vi "Recloser2.vi"() -> ()   [LabVIEW 2016]
uses:
  <vilib>/Utility/error.llb/DialogType.ctl
  <vilib>/Analysis/3filter.llb/Filter Passband Type.ctl
  <vilib>/FPGAPlugInAG/cRIO-9039 (Sync)/niLvFpga_Open_cRIO-9039 (Sync).vi
  <vilib>/rvi/interface/common/dynamic/niFpgaDynamicAddResources.vi
  <vilib>/addons/Electrical Power/Basic/Measurement/RMS (N Channels).vi
  <vilib>/measure/matone.llb/Extract Single Tone Information N Chan.vi
  <vilib>/Analysis/3filter.llb/Butterworth Filter (DBL).vi
  <vilib>/Utility/error.llb/Error Cluster From Error Code.vi
  <vilib>/rvi/errors/niLvFpgaAdjustHostInterfaceError.vi
  <vilib>/FPGAPlugInAG/Dynamic/niLvFpga_Abort_Dynamic.vi
  <vilib>/FPGAPlugInAG/Dynamic/niLvFpga_Close_Dynamic.vi
  <vilib>/rvi/interface/nirviOpenFPGA/nirviOpenFPGA.xnode
  FPGA Bitfiles/IntelliRupter2_FPGATarget.lvbitx
  <vilib>/rvi/interface/nirviReadWriteControl/nirviReadWriteControl.xnode
  <vilib>/rvi/interface/nirviMethod/nirviMethod.xnode
  <vilib>/rvi/interface/nirviCloseFPGA/nirviCloseFPGA.xnode
  <vilib>/addons/Electrical Power/Basic/NI_EP_Basic.lvlib
  <vilib>/measure/NI_MAPro.lvlib
  <vilib>/Analysis/NI_AALBase.lvlib
  NiFpgaLv.dll
  <vilib>/rvi/interface/Simulation/niFpgaSimulationCallBeginRW.vi
panel:
  out "VL Frequency":dbl
  in  "sampling freq: fs":dbl=1.0 format="%0.2f"
  out "magnitude difference":dbl
  out "frequency difference":dbl
  out "Phase difference":dbl
  out "average phase diff":dbl
  out "RMS values VR":dbl[](array[numeric])
  out "RMS values":dbl[](array[numeric])
  out "basic calc interval":u16=38
  out "half cycle (samples)":i32=96
  in  "Relay 8":bool
  in  "Tab Control":T1(tab)
  out "Waveform Chart":dynamicdata(graph)
  in  "samples per cycle":u16=192
  in  "Count(uSec)":u32=200
  in  "nominal frequency":u16=60
  in  "Magnitude Minimum":dbl=0.2
  in  "Magnitude difference level":dbl=0.1
  in  "Phase difference level":dbl=5.0
  in  "Frequency difference level":dbl=0.2
  out "VL Waveforms":waveform(sgl)[](graph)
  out "VR Waveforms":waveform(sgl)[](graph)=[{"t0"=timestamp(3610675669.9739585 s since 1904-01-01), "dt"=0.20000000298023224, "Y"=[-0.0016827583, -0.007917404, -0.0050468445, -0.0023388863, 0.0048799515, 0.002254963, -0.00037002563, -0.012183189, -0.014897823, -0.01054287, -0.0016827583, -4.196167e-05, 0.00061416626, -0.0052924156, -0.0024199486, -0.0049643517, -0.0046362877, -0.0059485435, -0.01907444, -0.0046362877, 0.015311241, -0.00069856644, -0.0023388863, 0.0042238235, 0.006192684, 0.0002861023, 0.0015201569, -0.0010266304, 0.0002861023, 0.001926899, 0.00061416626, -0.0016827583, 0.0025053024, 0.0012702942, -0.0049643517, -0.0059485435, -0.0062766075, 0.0012702942], "attributes"=variant("channel"=variant(u16 4))}, {"t0"=timestamp(3610675669.9739585 s since 1904-01-01), "dt"=0.20000000298023224, "Y"=[-0.009230137, -0.0053753853, 0.001598835, 0.002254963, 0.002583027, 0.0002861023, -0.011527061, 0.013669491, -0.0046362877, -4.196167e-05, 0.001598835, -0.0049643517, 0.0009422302, -0.00603199, -0.0072612762, 0.0012702942, -0.0020108223, 0.0045518875, -0.0069332123, -0.000121593475, 0.0012702942, -0.0010266304, 0.002254963, 0.0038957596, -0.0010266304, 0.014983177, -0.0020108223, -0.0010266304, 0.001926899, 0.001598835, -0.0016827583, -0.045763493, 0.0035672188, -0.003651619, -0.0049643517, -0.0072612762, -0.0052924156, -0.0030770302], "attributes"=variant("channel"=variant(u16 5))}, {"t0"=timestamp(3610675669.9739585 s since 1904-01-01), "dt"=0.20000000298023224, "Y"=[0.012684345, 0.0048799515, 0.0038957596, 0.00061416626, 0.0042238235, -0.0111989975, 0.005460739, -4.196167e-05, 0.0009422302, -0.00069856644, -0.003651619, 0.006520748, -0.0034050941, -0.009230137, 0.0002861023, -0.0023388863, 0.014396191, -0.003651619, -0.0047187805, -0.0016827583, -0.00037002563, -4.196167e-05, 0.0045518875, 0.0045518875, 0.022206783, 0.00061416626, 0.00061416626, 0.00061416626, 0.0009422302, -0.0010266304, -0.0030770302, -0.003979683, -0.0023388863, -0.0010266304, -0.012839794, 0.002254963, 0.0028338432, -0.0059485435], "attributes"=variant("channel"=variant(u16 6))}]
  in  "stop":bool
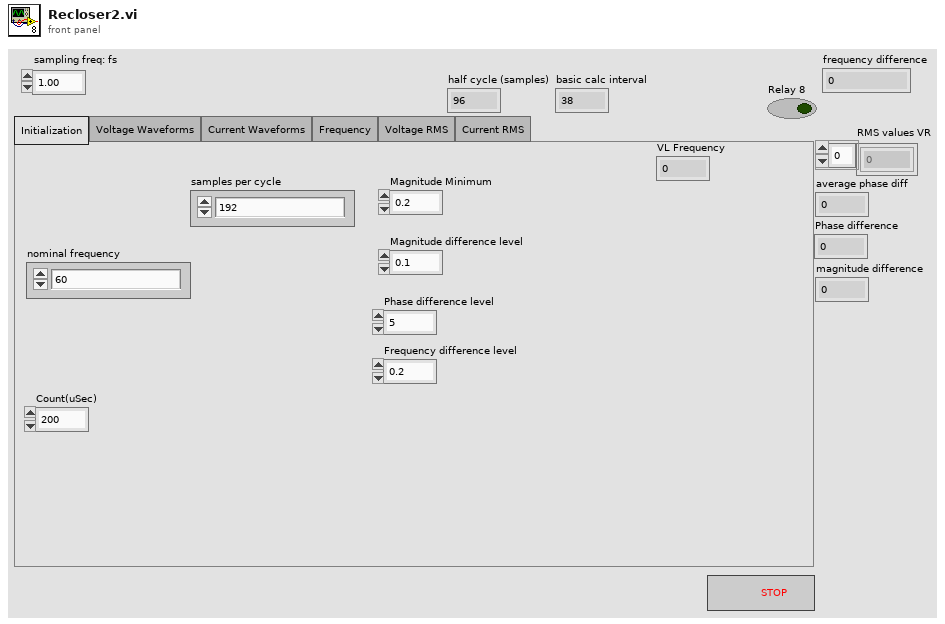
[diagram p1: front panel]
types:
  T1 = enum32{"Initialization", "Voltage Waveforms", "Current Waveforms", "Frequency", "Voltage RMS", "Current RMS"}
  T2 = enum16{"Va L", "Vb L", "Vc L", "Ia", "Ib", "Ic", "Va R", "Vb R", "Vc R"}[]
  T3 = typedef "DialogType.ctl" = u16
  T4 = typedef "NI_AALBase.lvlib/Filter Passband Type.ctl" = enum32{"Lowpass", "Highpass", "Bandpass", "Bandstop"}
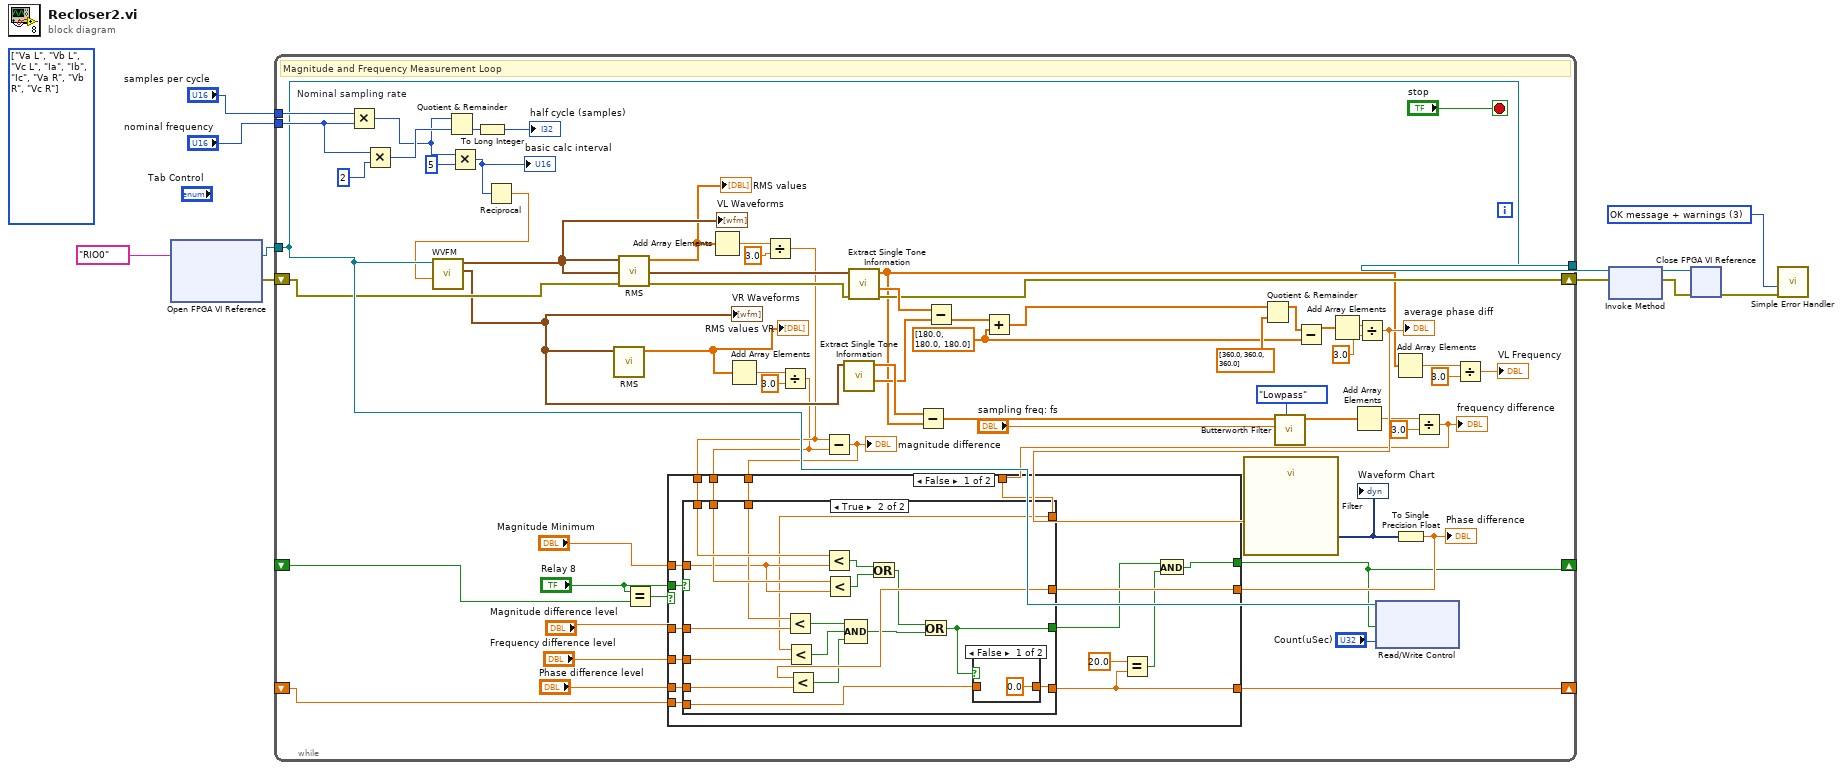
[diagram p0: block diagram]
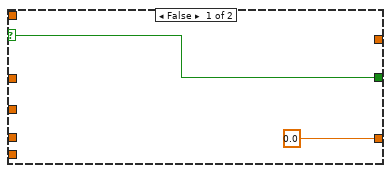
[diagram p2: hidden frame]
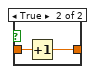
[diagram p3: hidden frame]
diagram:
  (unwired) T2 [enum."Va L", enum."Vb L", enum."Vc L", enum."Ia", enum."Ib", enum."Ic", enum."Va R", enum."Vb R", enum."Vc R"] items=["Va L", "Vb L", "Vc L", "Ia", "Ib", "Ic", "Va R", "Vb R", "Vc R"] ("Enum")
  w10 = T3 3 items=["no dialog", "OK message", "continue or stop message", "OK message + warnings", "continue/stop + warnings"] ("type of dialog (OK msg:1)")
  n1 = xnode "Open FPGA VI Reference"("resource name"=tag "RIO0") -> ("FPGA VI Reference Out"=w3:refnum<k20>, "error out"=w4:errorcluster)  [unwired: 1 in]
  n2 = while {
    shift-right: [w60] -> w9
    shift-left: w4 -> [w62]
    tunnel: w3 -> [w65]
    tunnel: [w65] -> w8
    tunnel: "samples per cycle" -> [w72]
    tunnel: "nominal frequency" -> [w71]
    shift-right: [w19] -> _
    shift-left: _ -> [w18]
    shift-right: [w17] -> _
    shift-left: _ -> [w16]
    stop <- "stop" stop-if-true
    w43 = dbl[] [180.0, 180.0, 180.0] ("y")
    # "Magnitude and Frequency Measurement Loop"
    n3 = Multiply "Nominal sampling rate"(x=w72, y=w71) -> (x*y=w55:u16)
    n4 = Multiply(x=w71, y=2) -> (x*y=w69:i32)
    n5 = Quotient & Remainder(x=w55, y=w69) -> (floor(x/y)=w67:i32)  [unwired: 1 out]
    n6 = Multiply(x=w55, y=u16 5) -> (x*y=w59:u16)
    "basic calc interval" <- w59
    n7 = To Long Integer(number=w67) -> (32bit integer=→"half cycle (samples)":i32)
    n8 = Reciprocal(x=w59) -> (1/x=w58:dbl)
    n9 = call "WVFM.vi"("dt"=w58, "FPGA VI Reference In"=w65) -> ("VR array"=w49:waveform(sgl)[], "VL array"=w50:waveform(sgl)[])  [unwired: 7 in]
    "VL Waveforms" <- w50
    "VR Waveforms" <- w49
    n10 = call-poly <vilib>:"RMS.vi"("waveforms"=w49) -> ("RMS values"=w26:dbl[])  [unwired: 9 in, 1 out]
    "RMS values VR" <- w26
    n11 = call-poly <vilib>:"RMS.vi"("error in (no error)"=w62, "waveforms"=w50) -> ("error out"=w61:errorcluster, "RMS values"=w29:dbl[])  [unwired: 8 in]
    "RMS values" <- w29
    n12 = Equal?(x="Relay 8", y=w16) -> (x = y?=w22:bool)
    n13 = Add Array Elements(numeric array=w29) -> (sum=w28:dbl)
    n14 = Add Array Elements(numeric array=w26) -> (sum=w32:dbl)
    n15 = Divide(x=w28, y=3.0) -> (x/y=w24:dbl)
    n16 = Divide(x=w32, y=3.0) -> (x/y=w23:dbl)
    n17 = Subtract(x=w24, y=w23) -> (x-y=w25:dbl)
    "magnitude difference" <- w25
    n18 = call-poly <vilib>:"Extract Single Tone Information.vi"("time signals in"=w49) -> ("detected phases (deg)"=w45:dbl[], "detected frequencies"=w57:dbl[])  [unwired: 5 in, 4 out]
    n19 = call-poly <vilib>:"Extract Single Tone Information.vi"("error in (no error)"=w61, "time signals in"=w50) -> ("error out"=w60:errorcluster, "detected phases (deg)"=w64:dbl[], "detected frequencies"=w12:dbl[])  [unwired: 4 in, 3 out]
    n20 = Subtract(x=w57, y=w12) -> (x-y=w56:dbl[])
    n21 = Subtract(x=w64, y=w45) -> (x-y=w46:dbl[])
    n22 = Add(x=w46, y=w43) -> (x+y=w53:dbl[])
    n23 = Quotient & Remainder(x=w53, y=dbl[] [360.0, 360.0, 360.0]) -> (x-y*floor(x/y)=w47:dbl[])  [unwired: 1 out]
    n24 = call-poly <vilib>:"Butterworth Filter.vi"("filter type"=Filter_Passband_Type."Lowpass", "sampling freq: fs"="sampling freq: fs", "X"=w56) -> ("Filtered X"=w39:dbl[])  [unwired: 5 in, 1 out]
    n25 = Subtract(x=w47, y=w43) -> (x-y=w44:dbl[])
    n26 = Add Array Elements(numeric array=w44) -> (sum=w52:dbl)
    n27 = Add Array Elements(numeric array=w39) -> (sum=w34:dbl)
    n28 = Divide(x=w52, y=3.0 ("x")) -> (x/y=w42:dbl)
    "average phase diff" <- w42
    n29 = call "Filter"("Signal"=w42) -> ("Filtered Signal"=w37:dynamicdata)  [unwired: 9 in, 1 out]
    "Waveform Chart" <- w37
    n30 = Add Array Elements(numeric array=w12) -> (sum=w14:dbl)
    n31 = To Single Precision Float(number=w37) -> (single precision float=w35:sgl)
    "Phase difference" <- w35
    n32 = Divide(x=w34, y=3.0) -> (x/y=w30:dbl)
    "frequency difference" <- w30
    n33 = case shown="False" w22 {
      tunnel: "Relay 8" -> [w89 w114]
      tunnel: "Magnitude Minimum" -> [w88 _]
      tunnel: "Magnitude difference level" -> [w87 _]
      tunnel: "Frequency difference level" -> [w86 _]
      tunnel: "Phase difference level" -> [w85 _]
      tunnel: w35 -> [w84 _]
      tunnel: w30 -> [w83 _]
      tunnel: w25 -> [w82 _]
      tunnel: w24 -> [w81 _]
      tunnel: w23 -> [w80 _]
      tunnel: [w75 _] -> w19
      tunnel: w18 -> [w79 _]
      tunnel: [w76 w114] -> w17
      frame False {
        n34 = case shown="True" w89 {
          selector: w89 -> [w91 _]
          tunnel: w81 -> [_ w110]
          tunnel: w80 -> [_ w109]
          tunnel: w82 -> [_ w106]
          tunnel: w88 -> [_ w105]
          tunnel: w87 -> [_ w104]
          tunnel: w83 -> [_ w103]
          tunnel: w86 -> [_ w102]
          tunnel: w84 -> [_ w101]
          tunnel: w85 -> [_ w100]
          tunnel: [w91 w92] -> w74
          tunnel: [0.0 w94] -> w75
          tunnel: w79 -> [_ w93]
          frame False {
          }
          frame True {
            n35 = Less?(x=w106, y=w104) -> (x < y?=w96:bool)
            n36 = Less?(x=w103, y=w102) -> (x < y?=w99:bool)
            n37 = Less?(x=w101, y=w100) -> (x < y?=w98:bool)
            n38 = Less?(x=w110, y=w105) -> (x < y?=w108:bool)
            n39 = Less?(x=w109, y=w105) -> (x < y?=w107:bool)
            n40 = Compound Arithmetic op=AND(w96, w99, w98) -> (w97:bool)
            n41 = Or(x=w108, y=w107) -> (x .or. y?=w95:bool)
            n42 = Or(x=w95, y=w97) -> (x .or. y?=w92:bool)
            n43 = case shown="False" w92 {
              tunnel: [0.0 w113] -> w94
              tunnel: w93 -> [_ w112]
              frame False {
              }
              frame True {
                n44 = Increment(x=w112) -> (x+1=w113:dbl)
              }
            }
          }
        }
        n45 = Equal?(x=20.0, y=w75) -> (x = y?=w77:bool)
        n46 = And(x=w74, y=w77) -> (x .and. y?=w76:bool)
      }
      frame True {
      }
    }
    n47 = xnode "Read/Write Control"("FPGA VI Reference In"=w65, "Relay1"=w17, "Count(ticks)"="Count(uSec)") -> ()  [unwired: 1 in, 2 out]
    n48 = Divide(x=w14, y=3.0) -> (x/y=→"VL Frequency":dbl)
  }
  n49 = xnode "Invoke Method"("FPGA VI Reference In"=w8, "error in"=w9) -> ("FPGA VI Reference Out"=w7:refnum<k20>, "error out"=w6:errorcluster)
  n50 = xnode "Close FPGA VI Reference"("FPGA VI Reference In"=w7, "error in"=w6) -> ("error out"=w11:errorcluster)
  n51 = call <vilib>:"Simple Error Handler.vi"("type of dialog (OK msg:1)"=w10, "error in (no error)"=w11) -> ()  [unwired: 3 in, 5 out]
